vi "gyro_get_header.vi"(10 "csv path":path, 11 "all rows":string[][](array[string])) -> (3 "header out":T1)   [LabVIEW 2020]
uses:
  <vilib>/regexp/Match Regular Expression.xnode
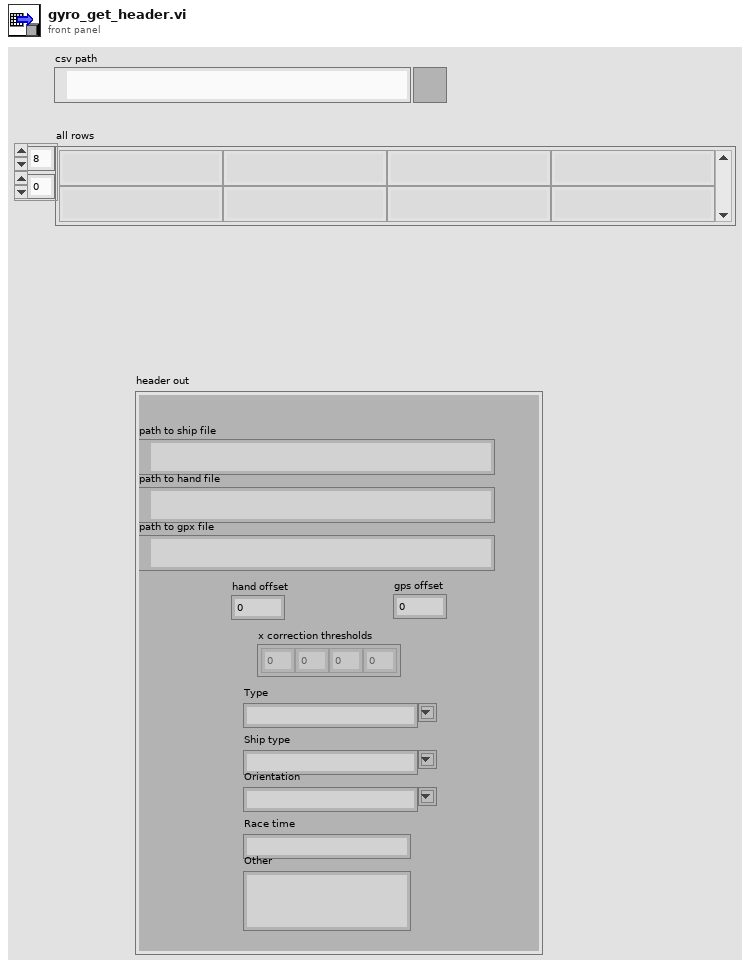
[diagram p1: front panel]
types:
  T1 = cluster{"path to ship file":path, "path to hand file":path, "path to gpx file":path, "hand offset":dbl, "gps offset":dbl, "x correction thresholds":i32[], "Type":string, "Ship type":string, "Orientation":string, "Race time":string, "Other":string}
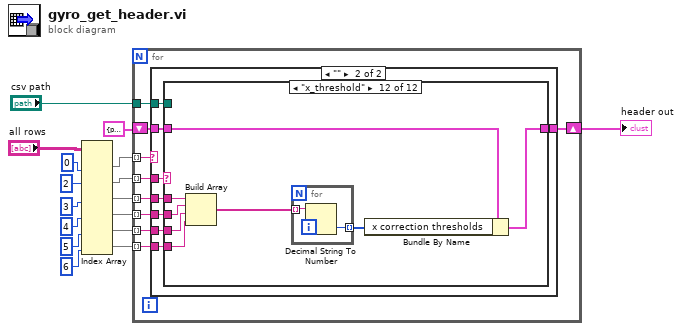
[diagram p0: block diagram]
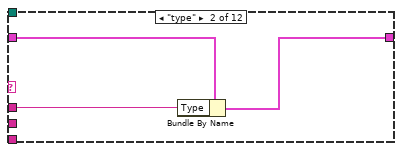
[diagram p4: hidden frame]
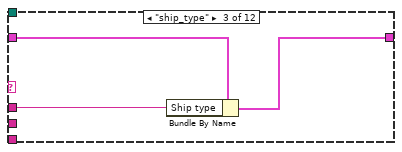
[diagram p5: hidden frame]
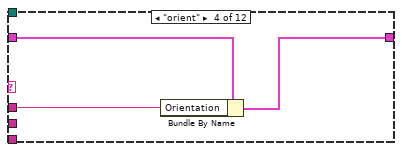
[diagram p6: hidden frame]
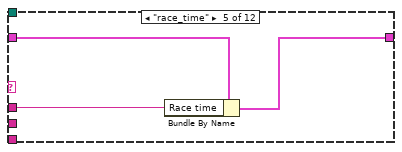
[diagram p7: hidden frame]
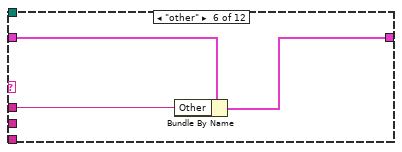
[diagram p8: hidden frame]
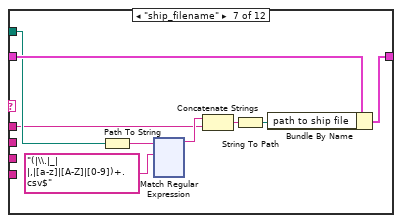
[diagram p9: hidden frame]
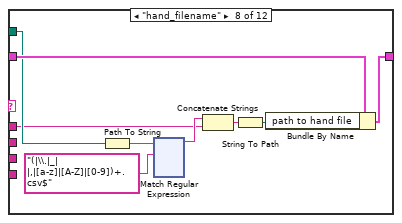
[diagram p10: hidden frame]
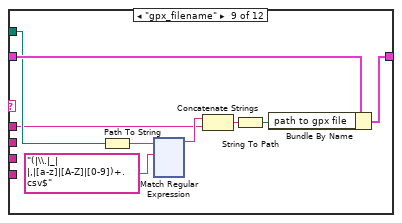
[diagram p11: hidden frame]
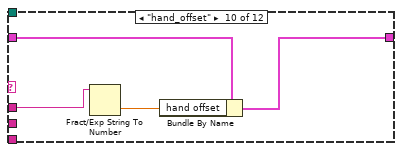
[diagram p12: hidden frame]
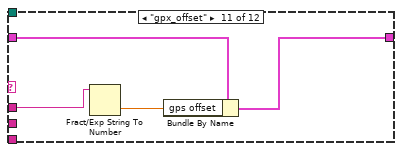
[diagram p13: hidden frame]
diagram:
  n1 = Index Array(array="all rows", index (col) #1=0 ("disabled index (col)"), index (col) #2=2 ("disabled index (row)"), index (col) #3=3 ("disabled index (row)"), index (col) #4=4 ("disabled index (row)"), index (col) #5=5 ("disabled index (row)"), index (col) #6=6 ("disabled index (row)")) -> (element #1=w16:string[], element #2=w15:string[], element #3=w14:string[], element #4=w4:string[], element #5=w3:string[], element #6=w2:string[])  [unwired: 6 in]
  n2 = for {
    tunnel: w16 -> [w25] mode=indexing
    tunnel: w15 -> [w24] mode=indexing
    tunnel: w14 -> [w23] mode=indexing
    shift-right: [w22] -> w9
    shift-left: T1 {"path to ship file"=path "", "path to hand file"=path "", "path to gpx file"=path "", "hand offset"=0.0, "gps offset"=0.0, "x correction thresholds"=[], "Type"="", "Ship type"="", "Orientation"="", "Race time"="", "Other"=""} ("header out") -> [w21]
    tunnel: "csv path" -> [w20]
    tunnel: w4 -> [w19] mode=indexing
    tunnel: w3 -> [w18] mode=indexing
    tunnel: w2 -> [w17] mode=indexing
    n3 = case shown="\"\"" w25 {
      tunnel: w24 -> [_ w34]
      tunnel: w23 -> [_ w33]
      tunnel: [w26 w32] -> w22
      tunnel: w21 -> [w26 w31]
      tunnel: w20 -> [_ w30]
      tunnel: w19 -> [_ w29]
      tunnel: w18 -> [_ w28]
      tunnel: w17 -> [_ w27]
      frame Default {
      }
      frame "" {
        n4 = case shown="\"x_threshold\"" w34 {
          tunnel: w33 -> [_ w38 w41 w44 w47 w50 w51 w174 w297 w420 w424 w432]
          tunnel: [w35 w37 w40 w43 w46 w49 w59 w182 w305 w423 w427 w435] -> w32
          tunnel: w31 -> [w35 w36 w39 w42 w45 w48 w58 w181 w304 w422 w426 w434]
          tunnel: w30 -> [_ _ _ _ _ _ w54 w177 w300 _ _ _]
          tunnel: w29 -> [_ _ _ _ _ _ _ _ _ _ _ w431]
          tunnel: w28 -> [_ _ _ _ _ _ _ _ _ _ _ w430]
          tunnel: w27 -> [_ _ _ _ _ _ _ _ _ _ _ w429]
          frame Default {
          }
          frame "type" {
            n5 = Bundle By Name(cluster=w36, "Type"=w38) -> (w37:T1)
          }
          frame "ship_type" {
            n6 = Bundle By Name(cluster=w39, "Ship type"=w41) -> (w40:T1)
          }
          frame "orient" {
            n7 = Bundle By Name(cluster=w42, "Orientation"=w44) -> (w43:T1)
          }
          frame "race_time" {
            n8 = Bundle By Name(cluster=w45, "Race time"=w47) -> (w46:T1)
          }
          frame "other" {
            n9 = Bundle By Name(cluster=w48, "Other"=w50) -> (w49:T1)
          }
          frame "ship_filename" {
            n10 = Path To String(path=w54) -> (string=w56:string)
            n11 = xnode "Match Regular Expression"("input string"=w56, "regular expression"="(|\\.|_| |,|[a-z]|[A-Z]|[0-9])+.csv$") -> ("before match"=w52:string)  [unwired: 4 in, 4 out]
            n12 = Concatenate Strings(w52, w51) -> (w53:string)
            n13 = String To Path(string=w53) -> (path=w57:path)
            n14 = Bundle By Name(cluster=w58, "path to ship file"=w57) -> (w59:T1)
          }
          frame "hand_filename" {
            n15 = Path To String(path=w177) -> (string=w179:string)
            n16 = xnode "Match Regular Expression"("input string"=w179, "regular expression"="(|\\.|_| |,|[a-z]|[A-Z]|[0-9])+.csv$") -> ("before match"=w175:string)  [unwired: 4 in, 4 out]
            n17 = Concatenate Strings(w175, w174) -> (w176:string)
            n18 = String To Path(string=w176) -> (path=w180:path)
            n19 = Bundle By Name(cluster=w181, "path to hand file"=w180) -> (w182:T1)
          }
          frame "gpx_filename" {
            n20 = Path To String(path=w300) -> (string=w302:string)
            n21 = xnode "Match Regular Expression"("input string"=w302, "regular expression"="(|\\.|_| |,|[a-z]|[A-Z]|[0-9])+.csv$") -> ("before match"=w298:string)  [unwired: 4 in, 4 out]
            n22 = Concatenate Strings(w298, w297) -> (w299:string)
            n23 = String To Path(string=w299) -> (path=w303:path)
            n24 = Bundle By Name(cluster=w304, "path to gpx file"=w303) -> (w305:T1)
          }
          frame "hand_offset" {
            n25 = Fract/Exp String To Number(string=w420) -> (number=w421:dbl)  [unwired: 3 in, 1 out]
            n26 = Bundle By Name(cluster=w422, "hand offset"=w421) -> (w423:T1)
          }
          frame "gpx_offset" {
            n27 = Fract/Exp String To Number(string=w424) -> (number=w425:dbl)  [unwired: 3 in, 1 out]
            n28 = Bundle By Name(cluster=w426, "gps offset"=w425) -> (w427:T1)
          }
          frame "x_threshold" {
            n29 = Build Array(w432, w431, w430, w429) -> (w428:string[])
            n30 = for {
              tunnel: w428 -> [w437] mode=indexing
              tunnel: [w436] -> w433 mode=indexing
              n31 = Decimal String To Number(string=w437) -> (number=w436:i32)  [unwired: 2 in, 1 out]
            }
            n32 = Bundle By Name(cluster=w434, "x correction thresholds"=w433) -> (w435:T1)
          }
        }
      }
    }
  }
  "header out" <- w9
